vi "Teleop.vi"(10 "Match Info":T3={"Autonomous Elapsed Seconds"=0.0, "TeleOp Elapsed Seconds"=0.0, "Disabled Elapsed Seconds"=0.0, "Visited Autonomous"=FALSE, "Visited TeleOp"=FALSE, "Visited Disabled"=FALSE, "Autonomous Settings"={"Autonomous Style"=enum."Independent", "VI Refnum"=refnum}}, 11 "Call Context":T4) -> ()   [LabVIEW 2011]
doc: "This VI is called for each TeleOp packet received from the DS where the robot is not disabled. It is often used to read from the joysticks and update I/O or to update setpoints for timed control loops. It should complete and return within 20 milliseconds or it may miss DS packets."
uses:
  <vilib>/Rock Robotics/WPI/DriverStation/WPI_DriverStationDerivedRobotMode.ctl
  <vilib>/Rock Robotics/WPI/DriverStation/WPI_DriverStationMatch Info.ctl
  <vilib>/Rock Robotics/WPI/Solenoid/WPI_SolenoidValue.ctl
  Robot Global Data.vi
  <vilib>/Rock Robotics/WPI/Solenoid/WPI_SolenoidSetEnum.vi
panel:
  in  "Kick Sonar":bool
  out "Pitch Gyro":dbl(knob) scale=-180.0..180.0
  in  "Dr1: Fetch":bool=TRUE
  in  "Dr10: Sensor Reset":bool
  out "Personality":string
  out "Auto Targeting ?":bool
  out "Angular Rate":dbl(knob) scale=0.0..400.0
  out "Distance Commanded":dbl
  out "Bridge Up":bool
  out "Bridge Down":bool
  in  "Slow Turret Div":dbl(knob)=5.060526308452546 scale=1.0..10.0
  out "Turret Stable?":bool
  out "Turret In Tol?":bool
  out "Use Turret Bumps":bool
  out "Turret Bumps":i64
  in  "RPM Bump Quanta":i64=40
  out "RPM Bumps":i64
  in  "Use Image for Distance ?":bool=TRUE
  out "Target Angle":dbl
  out "Target Distance":dbl
  out "RPM Stable?":bool
  out "Turret Home":bool
  out "Trigger":dbl(graph)
  in  "LowerLimit (v)":dbl(knob)=2.51198423272506 scale=0.0..5.0
  out "Meter":dbl(knob) scale=-0.1..0.1
  out "Ball Count":dbl
  out "State":T1
  in  "Gear":u16(ring)=1 items=["HIGH", "LOW"]
  in  "Use Distance?":bool=TRUE
  in  "Manual Distance":dbl=17.0
  out "BB B":bool
  out "PRIME":bool
  out "BB A/B":bool
  out "INTAKE":bool
  out "Turret Yaw":dbl(knob)=-0.7936798322703851 scale=-210.0..60.0
  out "Avg Wheel Encoder":dbl
  out "RPM Control Response":cluster{"RPM Control 2":dbl, dbl}(graph)
  out "Target Info":T2(array[cluster])
  out "RPM High":bool
  out "RPM Low":bool
  out "1 RPM":bool
  out "5 RPM":bool
  out "2 RPM":bool
  out "8 RPM":bool
  out "7 RPM":bool
  out "6 RPM":bool
  out "4 RPM":bool
  out "3 RPM":bool
  out "Ball Speed":dbl
  in  "Falling Edge":bool
  in  "Rising Edge":bool
  in  "Distance (in)":dbl
  out "speed (ft/s)":dbl
  in  "Shooter RPM Control":dbl(knob) scale=0.0..4000.0
  out "RPM In Tol?":bool
  out "Shooter RPM":dbl(knob) scale=0.0..4000.0
  out "Right Wheel Encoder":dbl
  out "Left Wheel Encoder":dbl
  out "Robot Gyro":dbl(knob) scale=-180.0..180.0
  # "Ball Launch Speed Sense"
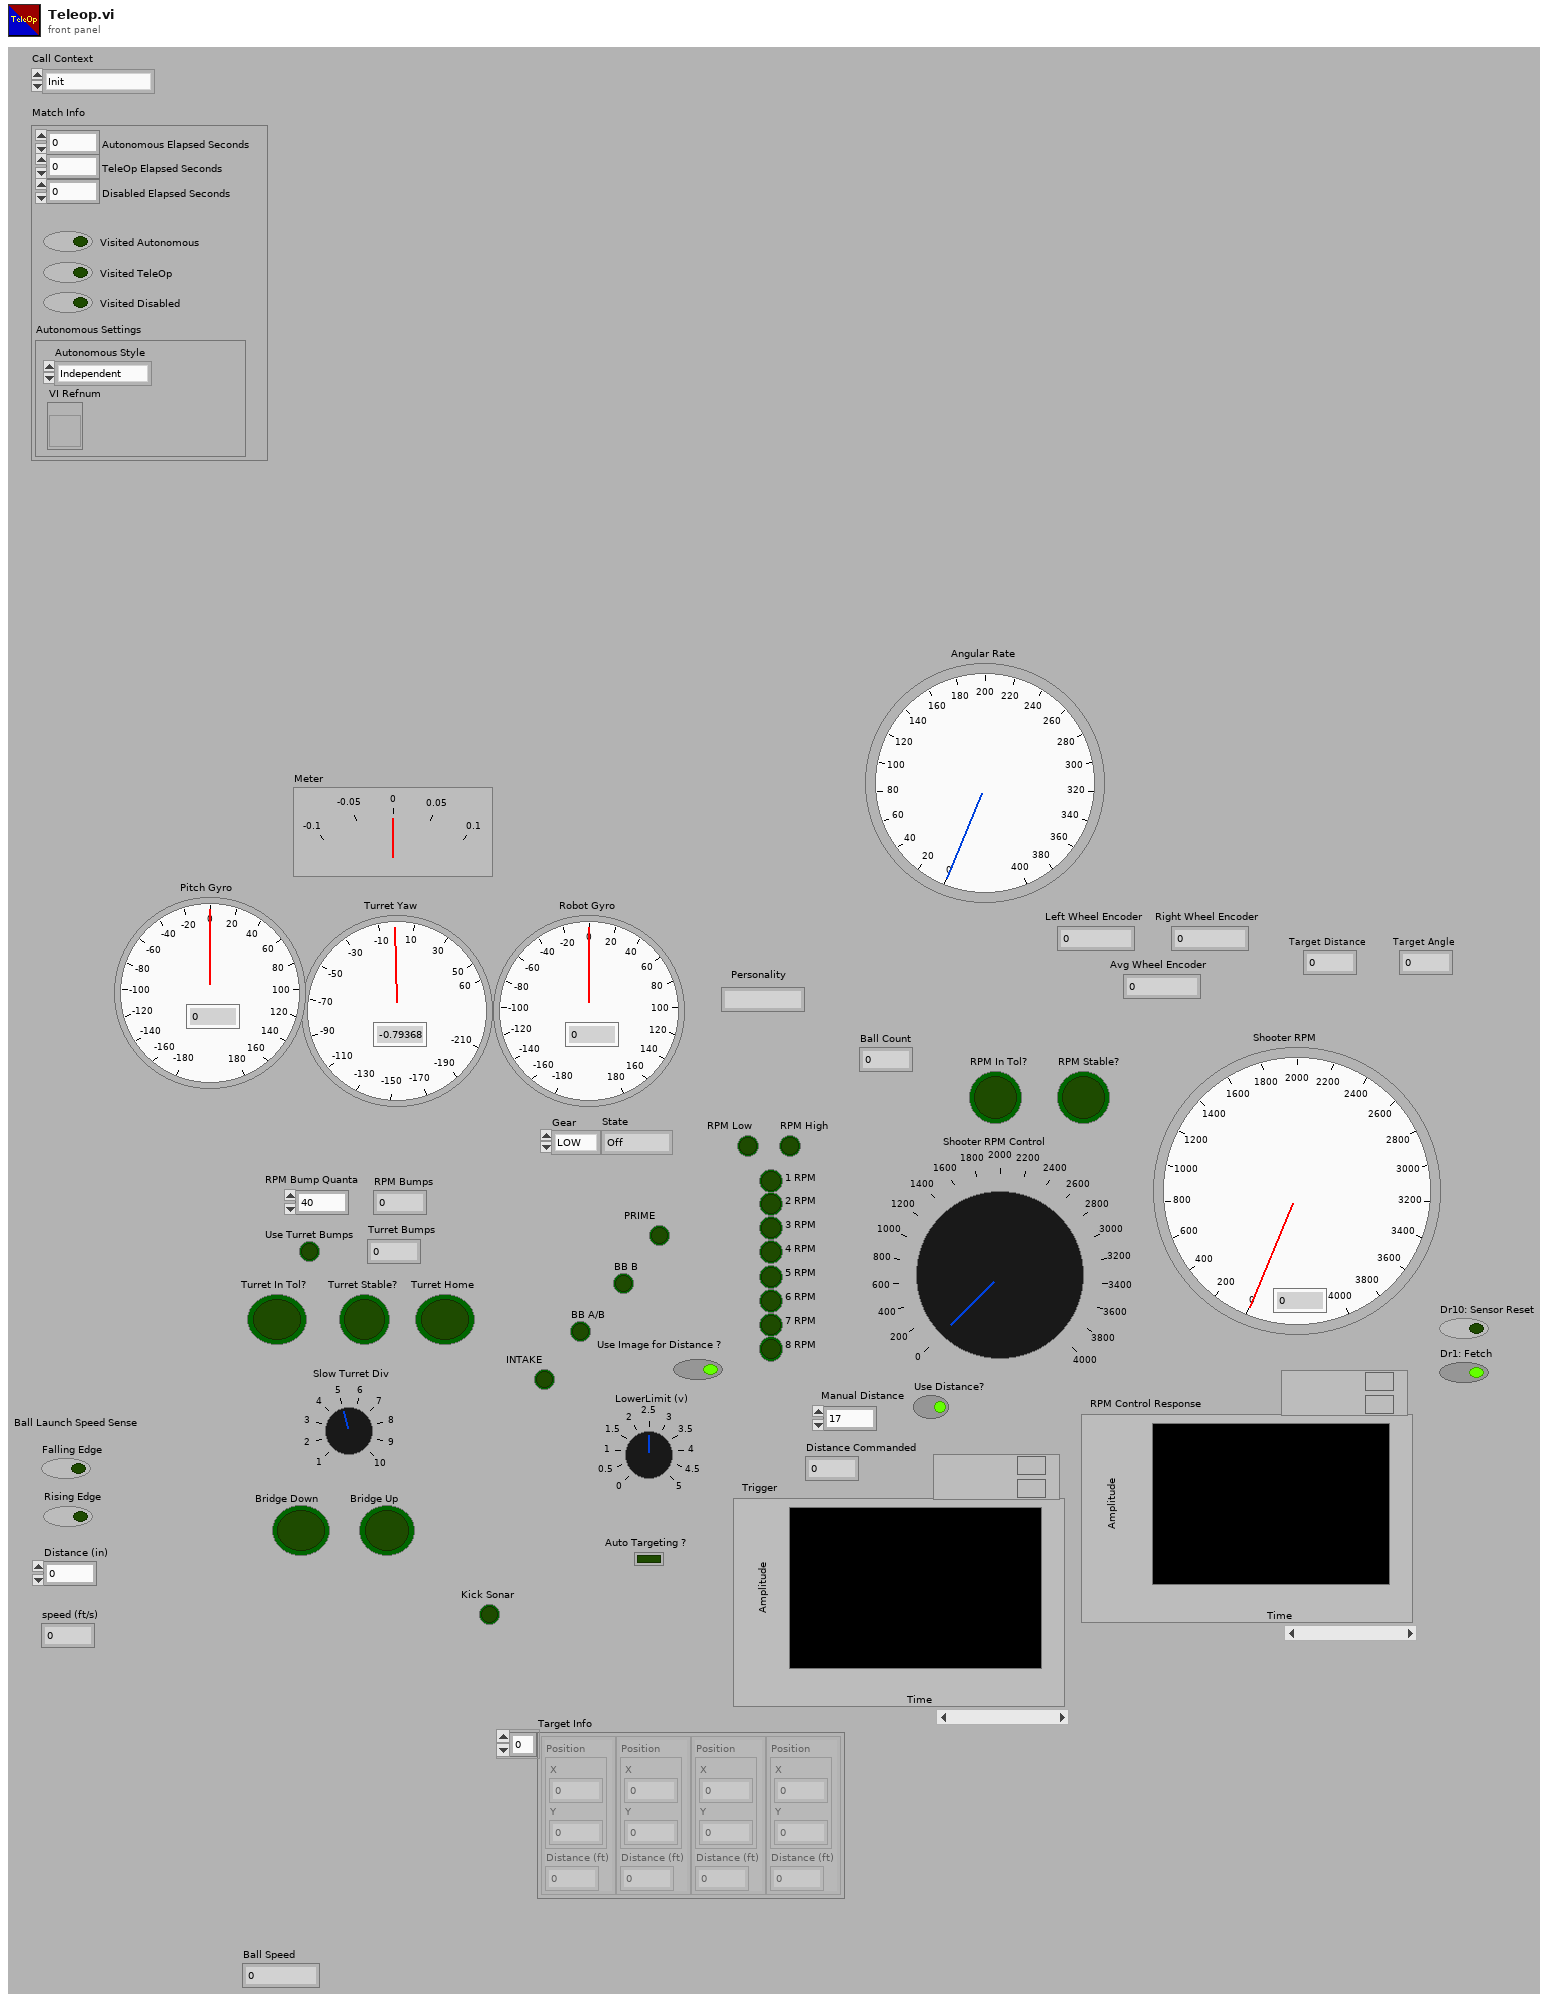
[diagram p1: front panel]
types:
  T1 = typedef "WPI_SolenoidValue.ctl" = enum16{"Off", "On", "Forward", "Reverse"}
  T2 = cluster{"Position":cluster{"X":dbl, "Y":dbl}, "Distance (ft)":dbl}[]
  T3 = typedef "WPI_DriverStationMatch Info.ctl" = cluster{"Autonomous Elapsed Seconds":dbl, "TeleOp Elapsed Seconds":dbl, "Disabled Elapsed Seconds":dbl, "Visited Autonomous":bool, "Visited TeleOp":bool, "Visited Disabled":bool, "Autonomous Settings":cluster{"Autonomous Style":enum16{"Iterative", "Independent"}, "VI Refnum":refnum<vi>}}
  T4 = typedef "WPI_DriverStationDerivedRobotMode.ctl" = enum16{"Init", "Execute", "Stop"}
  T5 = typedef "WPI_GyroDevRef.ctl" = cluster{"DevStatus":errorcluster, "Analog Module":T6, "Analog Channel":T7, "Offset":dbl, "Gain (VoltsPerDegree/Second)":dbl}
  T6 = typedef "FPGA_TypedefAnalogModule.ctl" = enum16{"Analog Module 1", "Analog Module 2"}
  T7 = typedef "FPGA_AIChannel.ctl" = enum8{"AI 1", "AI 2", "AI 3", "AI 4", "AI 5", "AI 6", "AI 7", "AI 8", "Invalid"}
  T8 = typedef "WPI_EncoderDevRef.ctl" = cluster{"DevStatus":errorcluster, "EncoderIndex":T9, "CounterIndex":T10, "DistancePerCount":dbl, "Decoding Type":T11}
  T9 = typedef "FPGA_EncoderIdx.ctl" = enum8{"Enc 0", "Enc 1", "Enc 2", "Enc 3", "Invalid"}
  T10 = typedef "FPGA_CounterCtrSystemIndex.ctl" = enum8{"Ctr 0", "Ctr 1", "Ctr 2", "Ctr 3", "Ctr 4", "Ctr 5", "Ctr 6", "Ctr 7", "Invalid"}
  T11 = typedef "WPI_EncoderType.ctl" = enum16{"1x", "2x", "4x"}
  T12 = typedef "WPI_JoystickDevRef.ctl" = cluster{"Device":T13}
  T13 = typedef "WPI_JoystickDeviceEnum.ctl" = enum16{"USB 1", "USB 2", "USB 3", "USB 4", "Kinect 1", "Kinect 2"}
  T14 = typedef "WPI_JoystickButtonState.ctl" = cluster{"Button 1":bool, "Button 2":bool, "Button 3":bool, "Button 4":bool, "Button 5":bool, "Button 6":bool, "Button 7":bool, "Button 8":bool, "Button 9":bool, "Button 10":bool, "Button 11":bool, "Button 12":bool}
  T15 = cluster{"axis 1 (x)":dbl, "axis 2 (y)":dbl, "axis 3 (throttle)":dbl, "axis 4":dbl, "axis 5":dbl, "axis 6":dbl}
  T16 = typedef "WPI_DigitalInputDevRef.ctl" = cluster{"DevStatus":errorcluster, "DIO Channel":T17, "Digital Module":T18}
  T17 = typedef "FPGA_DIOChannel.ctl" = enum8{"DIO 1", "DIO 2", "DIO 3", "DIO 4", "DIO 5", "DIO 6", "DIO 7", "DIO 8", "DIO 9", "DIO 10", "DIO 11", "DIO 12", "DIO 13", "DIO 14", "Invalid"}
  T18 = typedef "FPGA_TypedefDigitalModule.ctl" = enum16{"Digital Module 1", "Digital Module 2"}
  T19 = typedef "WPI_AnalogChannelDevRef.ctl" = cluster{"DevStatus":errorcluster, "Analog Module":T6, "Analog Channel":T7}
  T20 = typedef "FPGA_AnalogTriggerDevRef.ctl" = cluster{"DevStatus":errorcluster, "AnalogTriggerIndex":T21}
  T21 = typedef "FPGA_AnalogTriggerIndex.ctl" = enum8{"Trig 0", "Trig 1", "Trig 2", "Trig 3", "Trig 4", "Trig 5", "Trig 6", "Trig 7", "Invalid"}
  T22 = cluster{"Shooter RPM Control":dbl, "Shooter RPM Response":dbl}
  T23 = typedef "WPI_SolenoidDevRef.ctl" = cluster{"DevStatus":errorcluster, "Solenoid Module":T24, "Forward Solenoid Channel":T25, "Reverse Solenoid Channel":T25}
  T24 = typedef "FPGA_TypedefSolenoidModule.ctl" = enum16{"Solenoid Module 1", "Solenoid Module 2"}
  T25 = typedef "WPI_SolenoidChannel.ctl" = enum8{"Solenoid 1", "Solenoid 2", "Solenoid 3", "Solenoid 4", "Solenoid 5", "Solenoid 6", "Solenoid 7", "Solenoid 8", "Invalid"}
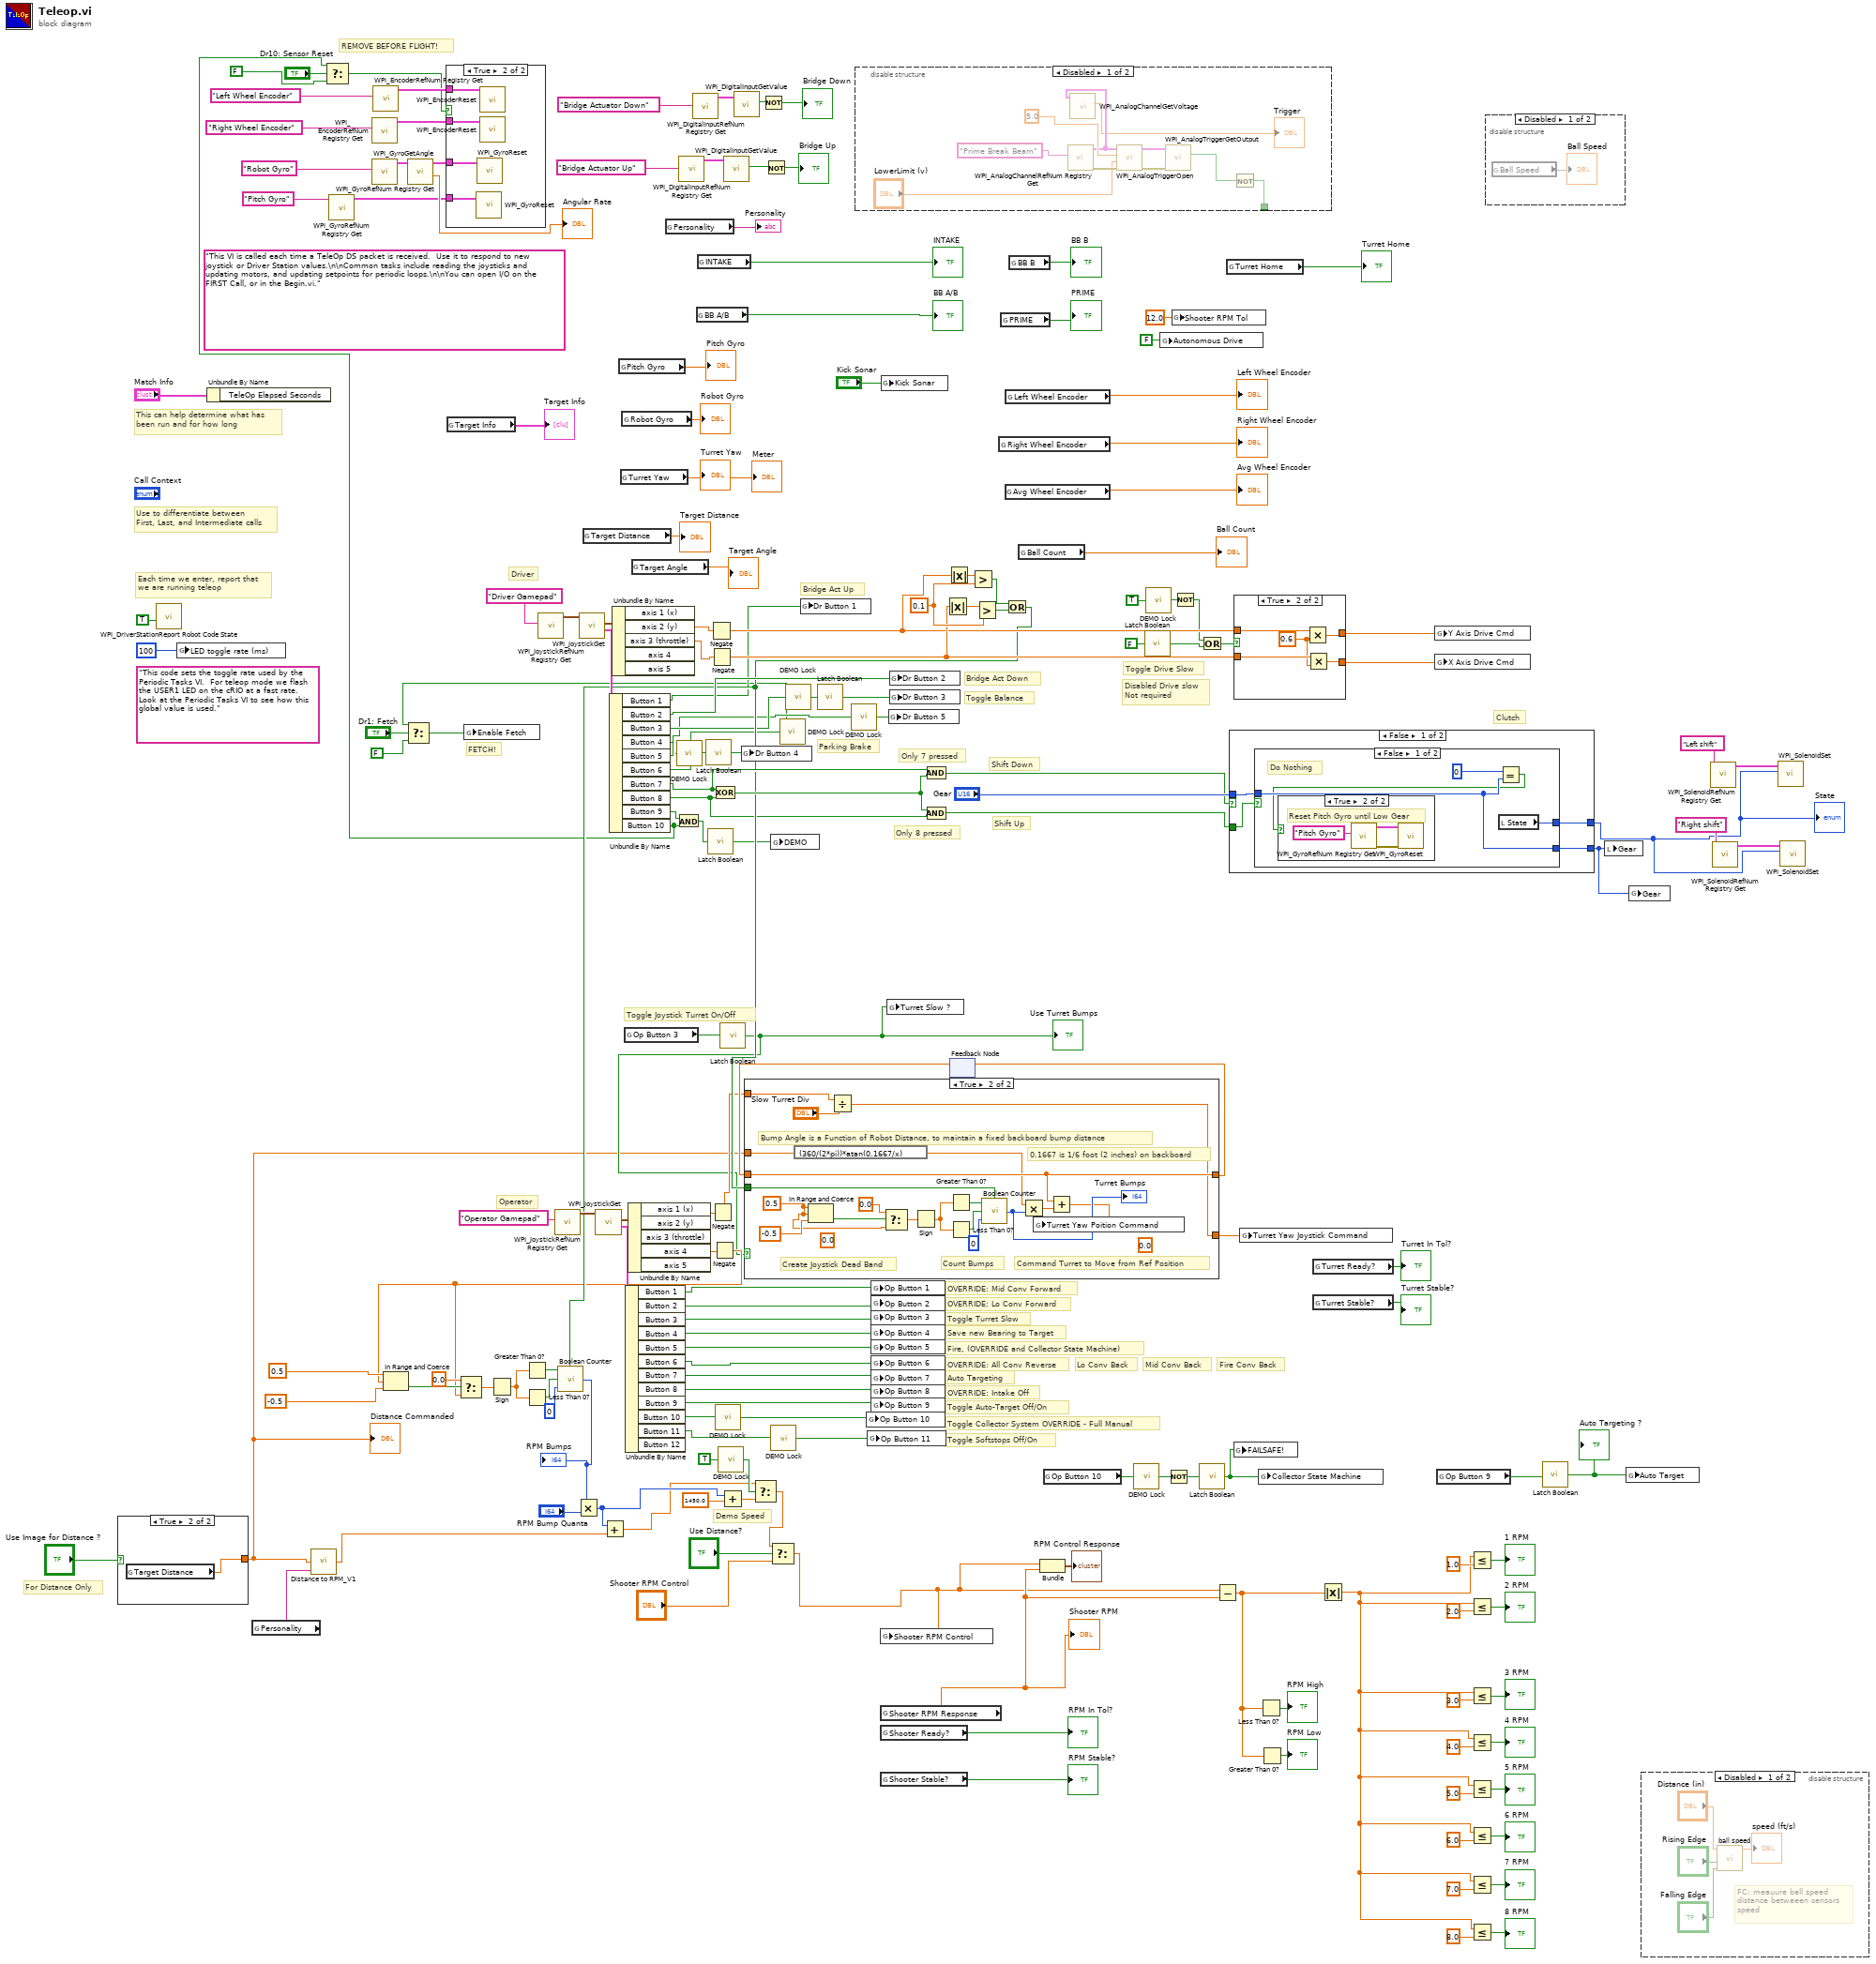
[diagram p0: block diagram]
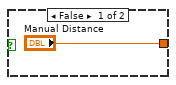
[diagram p2: hidden frame]
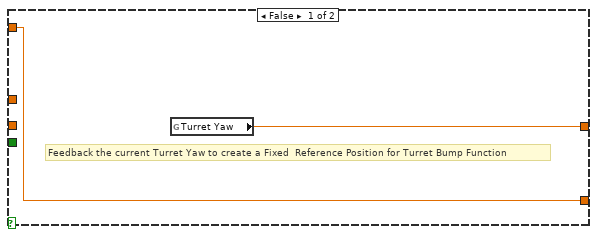
[diagram p3: hidden frame]
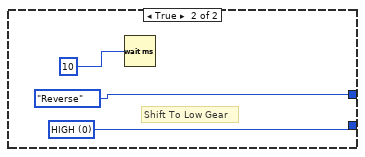
[diagram p7: hidden frame]
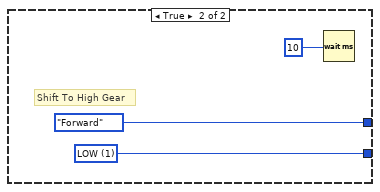
[diagram p8: hidden frame]
diagram:
  w94 = 0.1 ("y")
  (unwired) "This code sets the toggle rate used by the Periodic Tasks VI.  For teleop mode we flash the USER1 LED on the cRIO at a fast rate.  Look at the Periodic Tasks VI to see how this global value is used."
  (unwired) "This VI is called each time a TeleOp DS packet is received.  Use it to respond to new joystick or Driver Station values.\n\nCommon tasks include reading the joysticks and updating motors, and updating setpoints for periodic loops.\n\nYou can open I/O on the FIRST Call, or in the Begin.vi."
  # "FETCH!"
  # "Disabled Drive slow\nNot required"
  # "Demo Speed"
  # "Toggle Balance"
  # "Toggle Turret Slow"
  # "Toggle Softstops Off/On"
  # "Parking Brake"
  # "For Distance Only"
  # "Toggle Drive Slow"
  # "Toggle Joystick Turret On/Off"
  # "Auto Targeting"
  # "Toggle Collector System OVERRIDE - Full Manual"
  # "Bridge Act Up"
  # "Bridge Act Down"
  # "Toggle Auto-Target Off/On"
  # "OVERRIDE: Intake Off"
  # "Fire Conv Back"
  # "OVERRIDE: All Conv Reverse"
  # "REMOVE BEFORE FLIGHT!"
  # "Clutch"
  # "Shift Down"
  # "Shift Up"
  # "Only 8 pressed"
  # "Only 7 pressed"
  # "Driver"
  # "Save new Bearing to Target"
  # "Lo Conv Back"
  # "OVERRIDE: Lo Conv Forward"
  # "Mid Conv Back"
  # "OVERRIDE: Mid Conv Forward"
  # "Fire, (OVERRIDE and Collector State Machine)"
  # "Operator"
  # "Each time we enter, report that\nwe are running teleop"
  # "Use to differentiate between\nFirst, Last, and Intermediate calls"
  # "This can help determine what has\nbeen run and for how long"
  n1 = case shown="True" "Use Image for Distance ?" {
    tunnel: ["Manual Distance" w181] -> w13
    frame False {
    }
    frame True {
      n2 = global read "Robot Global Data.vi" "Target Distance"() -> (w181:dbl)
    }
  }
  "Distance Commanded" <- w13
  n3 = call <vilib>:"WPI_DriverStationReport Robot Code State.vi"("TeleOp"=TRUE ("Autonomous")) -> ()  [unwired: 10 in, 1 out]
  n4 = global write "Robot Global Data.vi" "LED toggle rate (ms)"(u32 100 ("LED ms toggle rate")) -> ()
  n5 = Unbundle By Name("Match Info") -> ()  [unwired: 1 out]
  n6 = global read "Robot Global Data.vi" "Personality"() -> (w10:string)
  n7 = call "Distance to RPM_V1.vi"("Personality"=w10, "Target Distance"=w13) -> ("Shooter RPM Control"=w12:dbl)  [unwired: 3 in]
  n8 = call <vilib>:"WPI_GyroRefNum Registry Get.vi"("refnum name"="Pitch Gyro") -> ("GyroDevRef"=w6:T5)  [unwired: 9 in, 1 out]
  n9 = call <vilib>:"WPI_EncoderRefNum Registry Get.vi"("refnum name"="Right Wheel Encoder") -> ("EncoderDevRef"=w113:T8)  [unwired: 9 in, 1 out]
  n10 = call <vilib>:"WPI_GyroRefNum Registry Get.vi"("refnum name"="Robot Gyro") -> ("GyroDevRef"=w65:T5)  [unwired: 9 in, 1 out]
  n11 = call <vilib>:"WPI_EncoderRefNum Registry Get.vi"("refnum name"="Left Wheel Encoder") -> ("EncoderDevRef"=w114:T8)  [unwired: 9 in, 1 out]
  n12 = call <vilib>:"WPI_GyroGetAngle.vi"("GyroDevRef"=w65) -> ("Angular Rate"=→"Angular Rate":dbl, "GyroDevRef"=w64:T5)  [unwired: 7 in, 2 out]
  n13 = global read "Robot Global Data.vi" "Target Info"() -> (→"Target Info":T2)
  n14 = call <vilib>:"WPI_JoystickRefNum Registry Get.vi"("refnum name"="Driver Gamepad") -> ("JoystickDevRef"=w126:T12)  [unwired: 1 in, 9 out]
  n15 = call <vilib>:"WPI_JoystickRefNum Registry Get.vi"("refnum name"="Operator Gamepad") -> ("JoystickDevRef"=w173:T12)  [unwired: 1 in, 9 out]
  n16 = call <vilib>:"WPI_JoystickGet.vi"("JoystickDevRef"=w126) -> ("Buttons"=w125:T14, "Axes"=w128:T15)  [unwired: 1 in, 4 out]
  n17 = global read "Robot Global Data.vi" "Target Distance"() -> (→"Target Distance":dbl)
  n18 = call <vilib>:"WPI_JoystickGet.vi"("JoystickDevRef"=w173) -> ("Buttons"=w172:T14, "Axes"=w175:T15)  [unwired: 1 in, 4 out]
  n19 = Unbundle By Name(w125) -> ("Button 1"=w4:bool, "Button 2"=w106:bool, "Button 3"=w51:bool, "Button 4"=w41:bool, "Button 5"=w42:bool, "Button 6"=w43:bool, "Button 7"=w124:bool, "Button 8"=w49:bool, "Button 9"=w31:bool, "Button 10"=w2:bool)
  n20 = Select(t=w2, s="Dr10: Sensor Reset", f=FALSE) -> (s? t:f=w19:bool)
  n21 = case shown="True" w19 {
    tunnel: w114 -> [_ w185]
    tunnel: w113 -> [_ w184]
    tunnel: w64 -> [_ w183]
    tunnel: w6 -> [_ w182]
    frame False {
    }
    frame True {
      n22 = call <vilib>:"WPI_GyroReset.vi"("GyroDevRef"=w182) -> ()  [unwired: 9 in, 2 out]
      n23 = call <vilib>:"WPI_GyroReset.vi"("GyroDevRef"=w183) -> ()  [unwired: 9 in, 2 out]
      n24 = call <vilib>:"WPI_EncoderReset.vi"("EncoderDevRef"=w185) -> ()  [unwired: 9 in, 2 out]
      n25 = call <vilib>:"WPI_EncoderReset.vi"("EncoderDevRef"=w184) -> ()  [unwired: 9 in, 2 out]
    }
  }
  n26 = Unbundle By Name(w128) -> ("axis 2 (y)"=w109:dbl, "axis 3 (throttle)"=w110:dbl)  [unwired: 3 out]
  n27 = global read "Robot Global Data.vi" "Pitch Gyro"() -> (→"Pitch Gyro":dbl)
  n28 = global read "Robot Global Data.vi" "Turret Yaw"() -> (→"Turret Yaw" →"Meter":dbl)
  n29 = global read "Robot Global Data.vi" "Robot Gyro"() -> (→"Robot Gyro":dbl)
  n30 = global read "Robot Global Data.vi" "Op Button 3"() -> (w95:bool)
  n31 = Unbundle By Name(w172) -> ("Button 1"=w145:bool, "Button 2"=w144:bool, "Button 3"=w143:bool, "Button 4"=w142:bool, "Button 5"=w139:bool, "Button 6"=w141:bool, "Button 7"=w140:bool, "Button 8"=w138:bool, "Button 9"=w137:bool, "Button 10"=w39:bool, "Button 11"=w37:bool)  [unwired: 1 out]
  n32 = Unbundle By Name(w175) -> ("axis 1 (x)"=w76:dbl, "axis 4"=w100:dbl)  [unwired: 3 out]
  n33 = global read "Robot Global Data.vi" "Target Angle"() -> (→"Target Angle":dbl)
  n34 = global read "Robot Global Data.vi" "Personality"() -> (→"Personality":string)
  n35 = call "DEMO Lock.vi"("Input"=w41) -> ("Output"=w40:bool)
  n36 = And(x=w31, y=w2) -> (x .and. y?=w30:bool)
  n37 = call <vilib>:"WPI_DigitalInputRefNum Registry Get.vi"("refnum name"="Bridge Actuator Up") -> ("DigitalInputDevRef"=w73:T16)  [unwired: 9 in, 1 out]
  n38 = call <vilib>:"WPI_DigitalInputRefNum Registry Get.vi"("refnum name"="Bridge Actuator Down") -> ("DigitalInputDevRef"=w71:T16)  [unwired: 9 in, 1 out]
  n39 = global read "Robot Global Data.vi" "BB A/B"() -> (→"BB A/B":bool)
  n40 = global read "Robot Global Data.vi" "INTAKE"() -> (→"INTAKE":bool)
  n41 = call "Latch Boolean.vi"("Boolean Input"=w40) -> ("Boolean Output"=w53:bool)
  n42 = call "Latch Boolean.vi"("Boolean Input"=w30) -> ("Boolean Output"=w29:bool)
  n43 = Negate(x=w109) -> (-x=w90:dbl)
  n44 = Negate(x=w110) -> (-x=w92:dbl)
  n45 = Negate(x=w76) -> (-x=w75:dbl)
  n46 = Negate(x=w100) -> (-x=w77:dbl)
  n47 = In Range and Coerce(upper limit=0.5, x=w77, lower limit=-0.5) -> (In Range?=w86:bool)  [unwired: 1 out]
  n48 = Select(t=0.0, s=w86, f=w77) -> (s? t:f=w87:dbl)
  n49 = Sign(1:w87) -> (0:w104:dbl)
  n50 = Greater Than 0?(x=w104) -> (x > 0?=w103:bool)
  n51 = Less Than 0?(x=w104) -> (x < 0?=w102:bool)
  n52 = Exclusive Or(1:w49, 2:w124) -> (0:w123:bool)
  n53 = call "DEMO Lock.vi"("Input"=w39) -> ("Output"=w38:bool)
  n54 = call "DEMO Lock.vi"("Input"=TRUE) -> ("Output"=w35:bool)
  n55 = call "Latch Boolean.vi"("Boolean Input"=w95) -> ("Boolean Output"=w62:bool)
  "Use Turret Bumps" <- w62
  n56 = call <vilib>:"WPI_DigitalInputGetValue.vi"("DigitalInputDevRef"=w73) -> ("Value"=w69:bool)  [unwired: 8 in, 2 out]
  n57 = call <vilib>:"WPI_DigitalInputGetValue.vi"("DigitalInputDevRef"=w71) -> ("Value"=w70:bool)  [unwired: 8 in, 2 out]
  n58 = global write "Robot Global Data.vi" "Dr Button 4"(w53) -> ()
  n59 = Not(x=w70) -> (.not. x?=→"Bridge Down":bool)
  n60 = Not(x=w69) -> (.not. x?=→"Bridge Up":bool)
  n61 = global write "Robot Global Data.vi" "DEMO"(w29) -> ()
  n62 = call "DEMO Lock.vi"("Input"=w37) -> ("Output"=w36:bool)
  n63 = call "DEMO Lock.vi"("Input"=w43) -> ("Output"=w3:bool)
  n64 = Select(t=w3, s="Dr1: Fetch", f=FALSE) -> (s? t:f=w14:bool)
  n65 = global write "Robot Global Data.vi" "Enable Fetch"(w14) -> ()
  n66 = call "DEMO Lock.vi"("Input"=w51) -> ("Output"=w50:bool)
  n67 = global write "Robot Global Data.vi" "Dr Button 1"(w4) -> ()
  n68 = call "Latch Boolean.vi"("Boolean Input"=w50) -> ("Boolean Output"=w45:bool)
  n69 = call "DEMO Lock.vi"("Input"=w42) -> ("Output"=w44:bool)
  n70 = disable-structure shown="Disabled" {
    disable-tunnel: [w187 _] -> _
    frame Disabled {
      n71 = call <vilib>:"WPI_AnalogChannelRefNum Registry Get.vi"("refnum name"="Prime Break Beam") -> ("error out"=w195:errorcluster, "AIDeviceRef"=w189:T19)  [unwired: 9 in]
      n72 = call <vilib>:"WPI_AnalogChannelGetVoltage.vi"("AIDeviceRef"=w189) -> ("Voltage"=→"Trigger":dbl)  [unwired: 8 in, 2 out]
      n73 = call <vilib>:"WPI_AnalogTriggerOpen.vi"("error in (no error)"=w195, "LowerLimit (v)"="LowerLimit (v)", "UpperLimit (v)"=5.0, "AnalogTriggerSource"=w189) -> ("error out"=w194:errorcluster, "AnalogTriggerDevRef"=w193:T20)  [unwired: 6 in]
      n74 = call <vilib>:"WPI_AnalogTriggerGetOutput.vi"("error in (no error)"=w194, "AnalogTriggerDevRef"=w193) -> ("In Window"=w186:bool)  [unwired: 6 in, 3 out]
      n75 = Not(x=w186) -> (.not. x?=w187:bool)
    }
    frame Enabled {
    }
  }
  n76 = global write "Robot Global Data.vi" "Op Button 10"(w38) -> ()
  n77 = global write "Robot Global Data.vi" "Op Button 11"(w36) -> ()
  n78 = global write "Robot Global Data.vi" "Op Button 1"(w145) -> ()
  n79 = global write "Robot Global Data.vi" "Op Button 2"(w144) -> ()
  n80 = global write "Robot Global Data.vi" "Op Button 3"(w143) -> ()
  n81 = global write "Robot Global Data.vi" "Op Button 4"(w142) -> ()
  n82 = global write "Robot Global Data.vi" "Op Button 5"(w139) -> ()
  n83 = global write "Robot Global Data.vi" "Op Button 6"(w141) -> ()
  n84 = global write "Robot Global Data.vi" "Op Button 7"(w140) -> ()
  n85 = global write "Robot Global Data.vi" "Op Button 8"(w138) -> ()
  n86 = global write "Robot Global Data.vi" "Op Button 9"(w137) -> ()
  n87 = global read "Robot Global Data.vi" "Shooter RPM Response"() -> (w134:dbl)
  "Shooter RPM" <- w134
  n88 = global read "Robot Global Data.vi" "Shooter Ready?"() -> (→"RPM In Tol?":bool)
  n89 = global read "Robot Global Data.vi" "Shooter Stable?"() -> (→"RPM Stable?":bool)
  n90 = global write "Robot Global Data.vi" "Kick Sonar"("Kick Sonar") -> ()
  n91 = global write "Robot Global Data.vi" "Turret Slow ?"(w62) -> ()
  n92 = global write "Robot Global Data.vi" "Dr Button 5"(w44) -> ()
  n93 = global write "Robot Global Data.vi" "Dr Button 2"(w106) -> ()
  n94 = global write "Robot Global Data.vi" "Dr Button 3"(w45) -> ()
  n95 = And(x=w124, y=w123) -> (x .and. y?=w57:bool)
  n96 = And(x=w123, y=w49) -> (x .and. y?=w56:bool)
  n97 = Absolute Value(x=w92) -> (abs(x)=w93:dbl)
  n98 = Absolute Value(x=w90) -> (abs(x)=w91:dbl)
  n99 = feedback #1() -> (w83:dbl)  [unwired: 1 in]
  n100 = Greater?(x=w91, y=w94) -> (0:w98:bool)
  n101 = Greater?(x=w93, y=w94) -> (0:w99:bool)
  n102 = global read "Robot Global Data.vi" "Right Wheel Encoder"() -> (→"Right Wheel Encoder":dbl)
  n103 = global read "Robot Global Data.vi" "PRIME"() -> (→"PRIME":bool)
  n104 = global read "Robot Global Data.vi" "Avg Wheel Encoder"() -> (→"Avg Wheel Encoder":dbl)
  n105 = Or(x=w98, y=w99) -> (x .or. y?=w78:bool)
  n106 = call "Boolean Counter.vi"("Reset"=w78, "Initial Count"=i64 0, "Count Down"=w102, "Count Up"=w103) -> ("Count"=w80:i64)
  "RPM Bumps" <- w80
  n107 = Multiply(x=w80, y="RPM Bump Quanta") -> (x*y=w24:i64)
  n108 = Add(x=w24, y=w12) -> (x+y=w11:dbl)
  n109 = Add(x=w24, y=1450.0 ("t")) -> (x+y=w26:dbl)
  n110 = case shown="True" w62 {
    tunnel: [w196 w200] -> w96
    tunnel: w78 -> [_ w212]
    tunnel: w83 -> [_ w204]
    tunnel: [w197 w204] -> w84
    tunnel: w13 -> [_ w203]
    tunnel: w75 -> [w196 w198]
    frame False {
      # "Feedback the current Turret Yaw to create a Fixed  Reference Position for Turret Bump Function"
      n111 = global read "Robot Global Data.vi" "Turret Yaw"() -> (w197:dbl)
    }
    frame True {
      (unwired) 0.0 ("x")
      (unwired) 0.0 ("x")
      w201 = 0.5 ("upper limit")
      (unwired) 0.0 ("axis 1 (x)")
      # "Bump Angle is a Function of Robot Distance, to maintain a fixed backboard bump distance"
      # "Command Turret to Move from Ref Position"
      # "Count Bumps"
      # "Create Joystick Dead Band"
      # "0.1667 is 1/6 foot (2 inches) on backboard"
      n112 = expression code="(360/(2*pi))*atan(0.1667/x)"(w203) -> (w202:dbl)
      n113 = In Range and Coerce(upper limit=w201, x=w201, lower limit=-0.5) -> (In Range?=w206:bool)  [unwired: 1 out]
      n114 = Divide(x=w198, y="Slow Turret Div") -> (x/y=w200:dbl)
      n115 = Select(t=0.0 ("f"), s=w206, f=w201) -> (s? t:f=w207:dbl)
      n116 = Sign(1:w207) -> (0:w213:dbl)
      n117 = Greater Than 0?(x=w213) -> (x > 0?=w214:bool)
      n118 = Less Than 0?(x=w213) -> (x < 0?=w215:bool)
      n119 = call "Boolean Counter.vi"("Reset"=w212, "Initial Count"=i64 0, "Count Down"=w215, "Count Up"=w214) -> ("Count"=w211:i64)
      "Turret Bumps" <- w211
      n120 = Multiply(x=w202, y=w211) -> (x*y=w210:dbl)
      n121 = Add(x=w204, y=w210) -> (x+y=w209:dbl)
      n122 = global write "Robot Global Data.vi" "Turret Yaw Poition Command"(w209) -> ()
    }
  }
  n123 = Select(t=w11, s=w35, f=w26) -> (s? t:f=w28:dbl)
  n124 = Select(t=w28, s="Use Distance?", f="Shooter RPM Control") -> (s? t:f=w27:dbl)
  n125 = global write "Robot Global Data.vi" "Shooter RPM Control"(w27) -> ()
  n126 = feedback-in #1(w84) -> ()
  n127 = global read "Robot Global Data.vi" "Left Wheel Encoder"() -> (→"Left Wheel Encoder":dbl)
  n128 = global read "Robot Global Data.vi" "BB B"() -> (→"BB B":bool)
  n129 = global read "Robot Global Data.vi" "Ball Count"() -> (→"Ball Count":dbl)
  n130 = Bundle("Shooter RPM Control"=w27, "Shooter RPM Response"=w134) -> (→"RPM Control Response":T22)  [unwired: 1 out]
  n131 = global read "Robot Global Data.vi" "Op Button 10"() -> (w21:bool)
  n132 = call "DEMO Lock.vi"("Input"=w21) -> ("Output"=w22:bool)
  n133 = call "Latch Boolean.vi"("Boolean Input"=FALSE) -> ("Boolean Output"=w46:bool)
  n134 = call "DEMO Lock.vi"("Input"=TRUE) -> ("Output"=w33:bool)
  n135 = global write "Robot Global Data.vi" "Autonomous Drive"(FALSE ("Autonomous Drive")) -> ()
  n136 = Not(x=w22) -> (.not. x?=w23:bool)
  n137 = global write "Robot Global Data.vi" "Shooter RPM Tol"(12.0 ("Shooter RPM Tol")) -> ()
  n138 = Not(x=w33) -> (.not. x?=w32:bool)
  n139 = Or(x=w32, y=w46) -> (x .or. y?=w47:bool)
  n140 = call "Latch Boolean.vi"("Boolean Input"=w23) -> ("Boolean Output"=w60:bool)
  n141 = Subtract(x=w27, y=w134) -> (x-y=w152:dbl)
  n142 = global read "Robot Global Data.vi" "Turret Home"() -> (→"Turret Home":bool)
  n143 = case shown="False" w57 {
    tunnel: w56 -> [w220 _]
    tunnel: [w219 WPI_SolenoidValue."Forward" ("Value")] -> w118
    tunnel: [w218 w232] -> w52
    tunnel: "Gear" -> [w217 _]
    frame False {
      n144 = case shown="False" w220 {
        tunnel: [w224 WPI_SolenoidValue."Reverse" ("Value")] -> w219
        tunnel: [w223 w229] -> w218
        tunnel: w217 -> [w223 _]
        frame False {
          # "Do Nothing"
          n145 = Equal?(x=u16 0, y=w223) -> (x = y?=w222:bool)
          n146 = case shown="True" w222 {
            frame False {
            }
            frame True {
              # "Reset Pitch Gyro until Low Gear"
              n147 = call <vilib>:"WPI_GyroRefNum Registry Get.vi"("refnum name"="Pitch Gyro") -> ("error out"=w226:errorcluster, "GyroDevRef"=w227:T5)  [unwired: 9 in]
              n148 = call <vilib>:"WPI_GyroReset.vi"("error in (no error)"=w226, "GyroDevRef"=w227) -> ()  [unwired: 8 in, 2 out]
            }
          }
          n149 = local read "State"() -> (w224:T1)
        }
        frame True {
          w229 = u16 0 items=["HIGH", "LOW"] ("Gear")
          # "Shift To Low Gear"
          n150 = Wait (ms)(milliseconds to wait=u32 10) -> ()  [unwired: 1 out]
        }
      }
    }
    frame True {
      w232 = u16 1 items=["HIGH", "LOW"] ("Gear")
      # "Shift To High Gear"
      n151 = Wait (ms)(milliseconds to wait=u32 10) -> ()  [unwired: 1 out]
    }
  }
  "State" <- w118
  n152 = case shown="True" w47 {
    tunnel: [w235 w239] -> w55
    tunnel: w90 -> [w235 w240]
    tunnel: [w234 w237] -> w54
    tunnel: w92 -> [w234 w238]
    frame False {
    }
    frame True {
      w236 = 0.6 ("y")
      n153 = Multiply(x=w240, y=w236) -> (x*y=w239:dbl)
      n154 = Multiply(x=w238, y=w236) -> (x*y=w237:dbl)
    }
  }
  n155 = global write "Robot Global Data.vi" "FAILSAFE!"(w60) -> ()
  n156 = global write "Robot Global Data.vi" "Turret Yaw Joystick Command"(w96) -> ()
  n157 = global write "Robot Global Data.vi" "Collector State Machine"(w60) -> ()
  n158 = Less Than 0?(x=w152) -> (x < 0?=→"RPM High":bool)
  n159 = Greater Than 0?(x=w152) -> (x > 0?=→"RPM Low":bool)
  n160 = global read "Robot Global Data.vi" "Turret Ready?"() -> (→"Turret In Tol?":bool)
  n161 = global read "Robot Global Data.vi" "Turret Stable?"() -> (→"Turret Stable?":bool)
  n162 = Absolute Value(x=w152) -> (abs(x)=w155:dbl)
  n163 = global write "Robot Global Data.vi" "Y Axis Drive Cmd"(w55) -> ()
  n164 = global write "Robot Global Data.vi" "X Axis Drive Cmd"(w54) -> ()
  n165 = global read "Robot Global Data.vi" "Op Button 9"() -> (w58:bool)
  n166 = Less Or Equal?(x=w155, y=1.0) -> (x <= y?=→"1 RPM":bool)
  n167 = Less Or Equal?(x=w155, y=2.0) -> (x <= y?=→"2 RPM":bool)
  n168 = Less Or Equal?(x=w155, y=3.0) -> (x <= y?=→"3 RPM":bool)
  n169 = Less Or Equal?(x=w155, y=4.0) -> (x <= y?=→"4 RPM":bool)
  n170 = Less Or Equal?(x=w155, y=5.0) -> (x <= y?=→"5 RPM":bool)
  n171 = Less Or Equal?(x=w155, y=6.0) -> (x <= y?=→"6 RPM":bool)
  n172 = Less Or Equal?(x=w155, y=7.0) -> (x <= y?=→"7 RPM":bool)
  n173 = Less Or Equal?(x=w155, y=8.0) -> (x <= y?=→"8 RPM":bool)
  n174 = disable-structure shown="Disabled" {
    frame Disabled {
      n175 = global read "Robot Global Data.vi" "Ball Speed"() -> (→"Ball Speed")
    }
    frame Enabled {
    }
  }
  n176 = call "Latch Boolean.vi"("Boolean Input"=w58) -> ("Boolean Output"=w59:bool)
  "Auto Targeting ?" <- w59
  n177 = local write "Gear"(w52) -> ()
  n178 = global write "Robot Global Data.vi" "Auto Target"(w59) -> ()
  n179 = global write "Robot Global Data.vi" "Gear"(w52) -> ()
  n180 = disable-structure shown="Disabled" {
    frame Disabled {
      # "FC: meauure ball speed\ndistance betweeen sensors\nspeed"
      n181 = call "ball speed.vi"("Falling Edge"="Falling Edge", "Rising Edge"="Rising Edge", "Distance (in)"="Distance (in)") -> ("speed (ft/s)"=→"speed (ft/s)":dbl)  [unwired: 8 in]
    }
    frame Enabled {
    }
  }
  n182 = call <vilib>:"WPI_SolenoidRefNum Registry Get.vi"("refnum name"="Left shift") -> ("SolenoidDevRef"=w119:T23)  [unwired: 9 in, 1 out]
  n183 = call <vilib>:"WPI_SolenoidRefNum Registry Get.vi"("refnum name"="Right shift") -> ("SolenoidDevRef"=w120:T23)  [unwired: 9 in, 1 out]
  n184 = call-poly <vilib>:"WPI_SolenoidSet.vi"("Value"=w118, "SolenoidDevRef"=w119) -> ()  [unwired: 8 in, 2 out]
  n185 = call-poly <vilib>:"WPI_SolenoidSet.vi"("Value"=w118, "SolenoidDevRef"=w120) -> ()  [unwired: 8 in, 2 out]
